vi "Wind Farm #2 Cluster.vi"() -> (0 "Cluster":T1)   [LabVIEW 2009]
doc: "This is the cluster for Wind Farm #2.\n\nAAL 9/09"
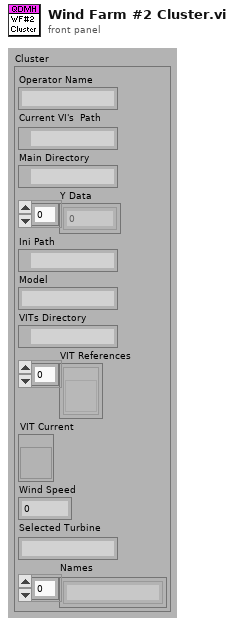
[diagram p1: front panel]
types:
  T1 = cluster{"Operator Name":string, "Current VI's  Path":path, "Main Directory":path, "Y Data":dbl[], "Ini Path":path, "Model":string, "VITs Directory":path, "VIT References":refnum<vi>[], "VIT Current":refnum<vi>, "Wind Speed":dbl, "Selected Turbine":string, "Names":string[]}
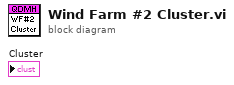
[diagram p0: block diagram]
diagram:
